vi "testCamera2.vi"() -> ()   [LabVIEW 2018]
uses:
  <vilib>/userdefined/High Color/IMAQdx.ctl
  vision/vision info 2.vi
  <vilib>/vision/driver/NI_Vision_Acquisition_Software.lvlib
  <resource>/objmgr/imaqdx.rc
panel:
  out "Image 2":T1(plugin-control)
  out "size(s)":i32
  out "Circles 2":cluster{"x":dbl, "y":dbl, "r":dbl}[](array[cluster])
  out "Circles":cluster{"x":dbl, "y":dbl, "r":dbl}[](array[cluster])
  out "Image":T1(plugin-control)
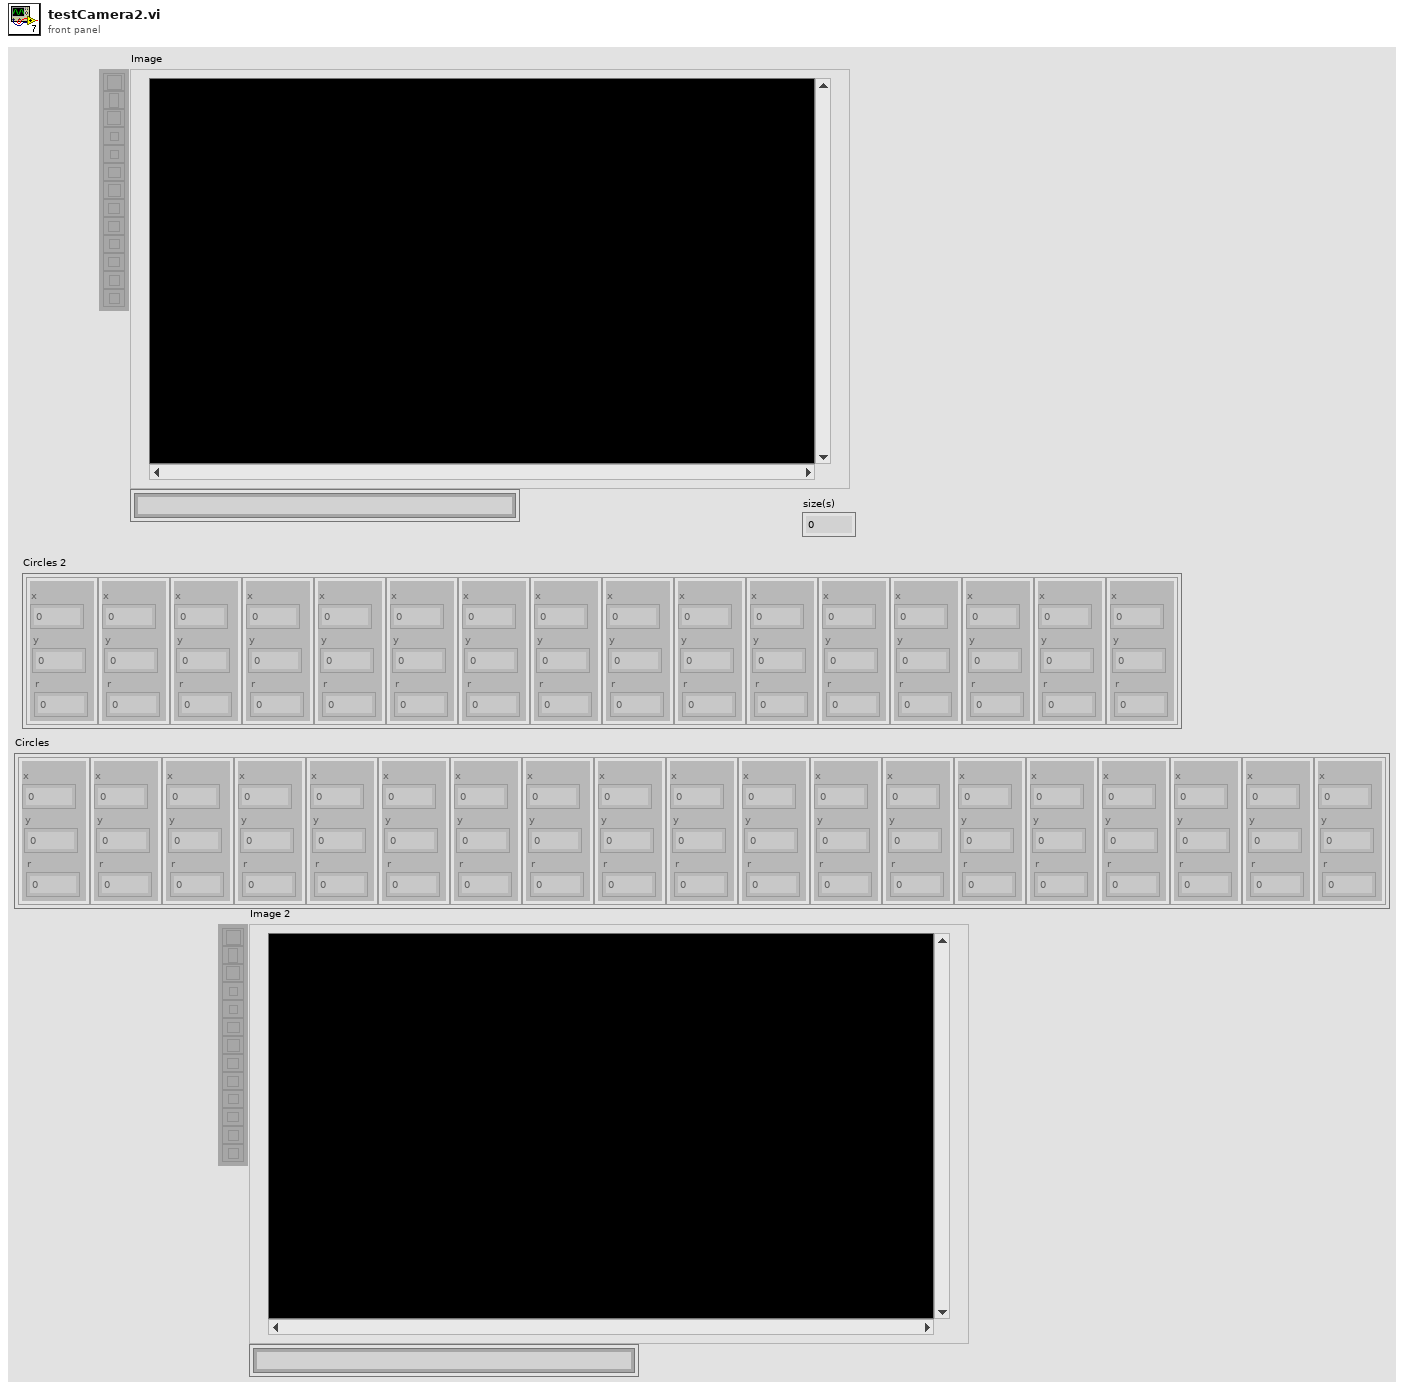
[diagram p1: front panel]
types:
  T1 = typedef "IMAQ Image.ctl" = refnum<image>
  T2 = typedef "IMAQdx.ctl" = refnum<k21>
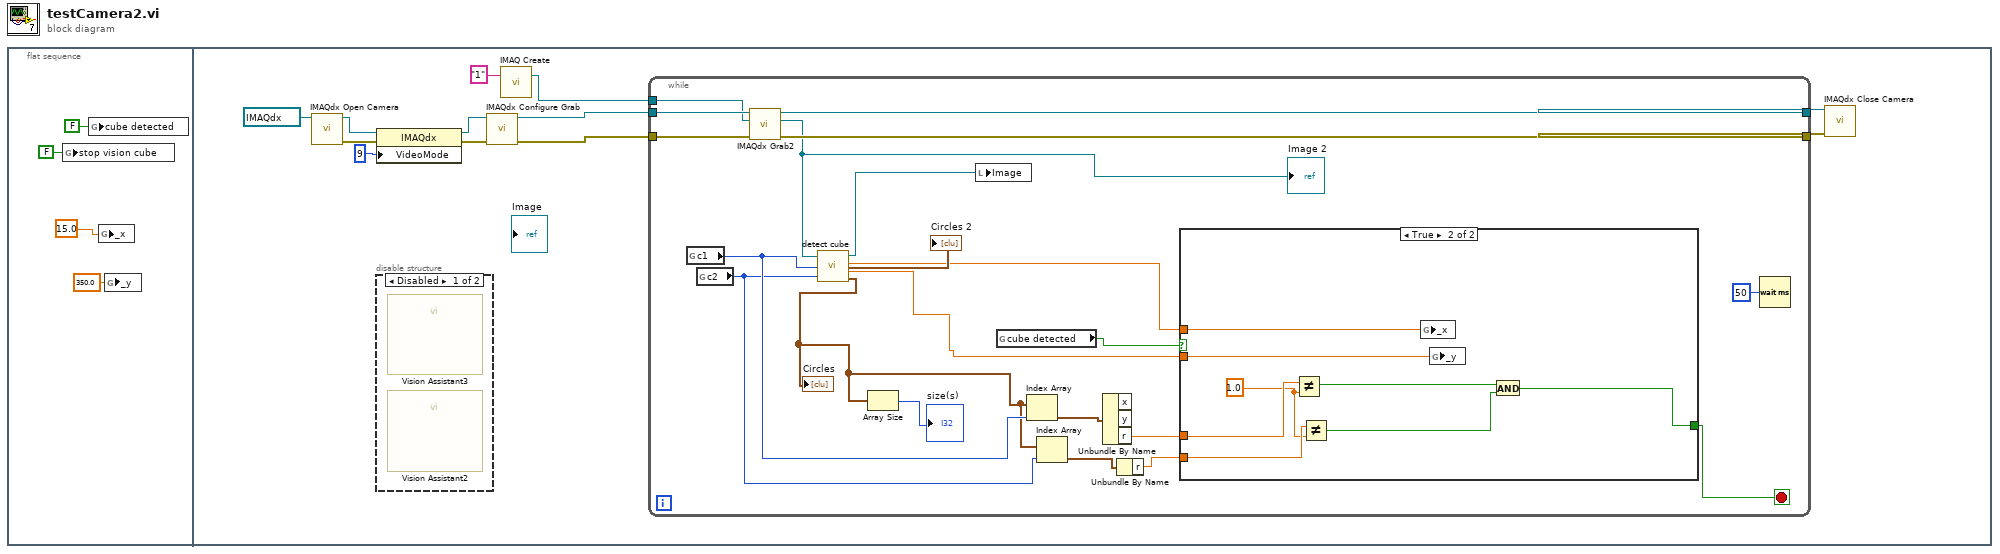
[diagram p0: block diagram]
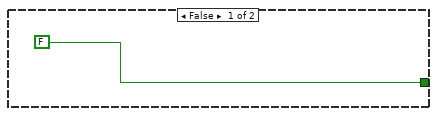
[diagram p3: hidden frame]
diagram:
  n1 = flat-sequence {
    frame #0 {
      n2 = global write "vision info 2.vi" "stop vision cube"(FALSE ("stop vision cube")) -> ()
      n3 = global write "vision info 2.vi" "cube detected"(FALSE ("cube detected")) -> ()
      n4 = global write "vision info 2.vi" "_x"(15.0 ("_x")) -> ()
      n5 = global write "vision info 2.vi" "_y"(350.0 ("_y")) -> ()
    }
    frame #1 {
      n6 = call <vilib>:"IMAQdx Open Camera.vi"("Session In"=T2 "cam0") -> ("error out"=w8:errorcluster, "Session Out"=w9:T2)  [unwired: 9 in]
      n7 = property class="IMAQdx"(reference=w9, error in=w8, "VideoMode"=u32 9) -> (reference out=w6:T2, error out=w7:errorcluster)
      n8 = disable-structure shown="Disabled" {
        frame Disabled {
          n9 = call "Vision Assistant3"() -> ()  [unwired: 26 in, 2 out]
          n10 = call "Vision Assistant2"() -> ()  [unwired: 26 in, 2 out]
        }
        frame Enabled {
        }
      }
      n11 = call <vilib>:"IMAQdx Configure Grab.vi"("error in"=w7, "Session In"=w6) -> ("error out"=w15:errorcluster, "Session Out"=w14:T2)  [unwired: 8 in]
      n12 = call "IMAQ Create"("Image Name"="1") -> ("New Image"=w12:T1)  [unwired: 4 in, 1 out]
      n13 = while {
        tunnel: w15 -> [w37]
        tunnel: w14 -> [w36]
        tunnel: [w35] -> w13
        tunnel: w12 -> [w34]
        tunnel: [w33] -> w10
        stop <- w17 stop-if-true
        n14 = global read "vision info 2.vi" "c1"() -> (w24:i8)
        n15 = global read "vision info 2.vi" "c2"() -> (w23:i8)
        n16 = call <vilib>:"IMAQdx Grab2.vi"("error in"=w37, "Image In"=w34, "Session In"=w36) -> ("error out"=w33:errorcluster, "Image Out"=w30:T1, "Session Out"=w35:T2)  [unwired: 5 in, 1 out]
        "Image 2" <- w30
        n17 = call "detect cube.vi"("Image 3"=w30, "c1"=w24, "c2"=w23) -> ("Image 4"=w31:T1, "_x"=w28:dbl, "_y"=w27:dbl, "Circles"=w22:cluster{"x":dbl, "y":dbl, "r":dbl}[], "Circles 2"=→"Circles 2":cluster{"x":dbl, "y":dbl, "r":dbl}[])
        "Circles" <- w22
        n18 = Array Size(array=w22) -> (size(s)=→"size(s)":i32)
        n19 = local write "Image"(w31) -> ()
        n20 = global read "vision info 2.vi" "cube detected"() -> (w25:bool)
        n21 = Index Array(array=w22, index=w24) -> (element=w21:cluster{"x":dbl, "y":dbl, "r":dbl})
        n22 = Index Array(array=w22, index=w23) -> (element=w20:cluster{"x":dbl, "y":dbl, "r":dbl})
        n23 = Unbundle By Name(w21) -> ("r"=w19:dbl)  [unwired: 2 out]
        n24 = Unbundle By Name(w20) -> ("r"=w18:dbl)
        n25 = case shown="True" w25 {
          tunnel: w28 -> [_ w46]
          tunnel: w27 -> [_ w45]
          tunnel: [FALSE ("stop vision cube") w39] -> w17
          tunnel: w19 -> [_ w44]
          tunnel: w18 -> [_ w43]
          frame False {
          }
          frame True {
            w42 = 1.0 ("y")
            n26 = Not Equal?(x=w44, y=w42) -> (x != y?=w40:bool)
            n27 = Not Equal?(x=w43, y=w42) -> (x != y?=w41:bool)
            n28 = global write "vision info 2.vi" "_x"(w46) -> ()
            n29 = global write "vision info 2.vi" "_y"(w45) -> ()
            n30 = And(x=w40, y=w41) -> (x .and. y?=w39:bool)
          }
        }
        n31 = Wait (ms)(milliseconds to wait=u32 50) -> ()  [unwired: 1 out]
      }
      n32 = call <vilib>:"IMAQdx Close Camera.vi"("error in"=w10, "Session In"=w13) -> ()  [unwired: 9 in, 1 out]
    }
  }
